vi "UDP_read_receive_buffer.vi"(6 "error in (no error)":errorcluster, 9 "connection ID":refnum<k16>) -> (0 "error out":errorcluster, 2 "Receive Buffer Size":u32, 3 "connection ID out":refnum<k16>)   [LabVIEW 2024]
doc: "This VI gets the receive buffer size for a given UDP socket connection."
uses:
  wsock32.dll
panel:
  in  "optlen":u32=4
  in  "optval: Rx Buffer Size":u32=8192
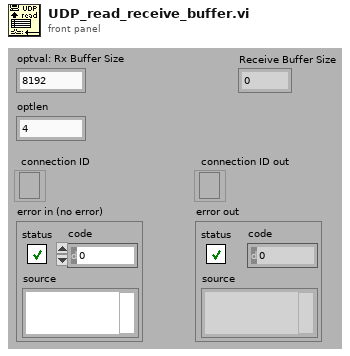
[diagram p1: front panel]
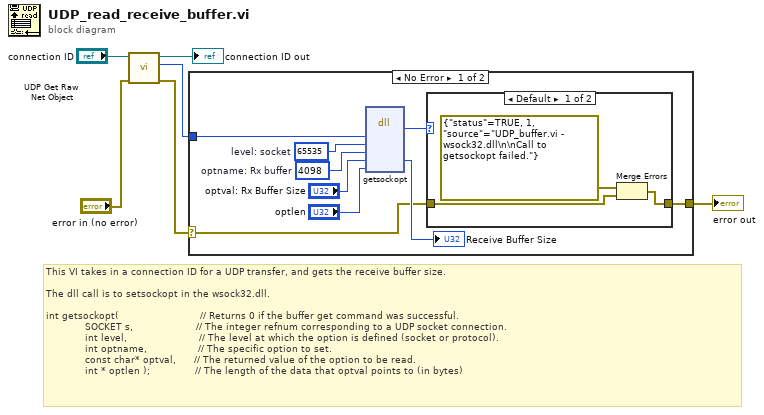
[diagram p0: block diagram]
diagram:
  # "This VI takes in a connection ID for a UDP transfer, and gets the receive buffer size.\n\nThe dll call is to setsockopt in the wsock32.dll.\n\nint getsockopt(                           // Returns 0 if the buffer get command was successful.\n             SOCKET s,                     // The integer refnum corresponding to a UDP socket connection.     \n             int level,                        // The level at which the option is defined (socket or protocol). \n             int optname,                 // The specific option to set.\n             const char* optval,      // The returned value of the option to be read.\n             int * optlen );               // The length of the data that optval points to (in bytes)"
  n1 = call <vilib>:"UDP Get Raw Net Object.vi"("error in (no error)"="error in (no error)", "connection ID"="connection ID") -> ("error out"=w6:errorcluster, "raw net object"=w3:u64, "connection ID out"=→"connection ID out":refnum<k16>)  [unwired: 7 in]
  n2 = case shown="No Error" w6 {
    selector: w6 -> [w7 w20]
    tunnel: [w12 w20] -> w2
    tunnel: w3 -> [w11 _]
    frame No Error {
      w14 = 4098  # optname: Rx buffer
      w15 = 65535  # level: socket
      n3 = dll-call lib="wsock32.dll" fn="getsockopt" ("Call Library Function")("socket"=w11, "protocol"=w15, "selector"=w14, "value"="optval: Rx Buffer Size", "size"="optlen") -> ("return type"=w13:i32, "value"=→"Receive Buffer Size":u32)  [unwired: 7 in, 2 out]
      n4 = case shown="Default" w13 {
        tunnel: [w18 w19] -> w12
        tunnel: w7 -> [w16 w19]
        frame Default {
          n5 = Merge Errors(cluster{"status":bool, i32, "source":string} {"status"=TRUE, 1, "source"="UDP_buffer.vi - wsock32.dll\n\nCall to getsockopt failed."} ("error out"), w16) -> (w18:errorcluster)
        }
        frame 0 {
        }
      }
    }
    frame Error {
    }
  }
  "error out" <- w2
